vi "ParameterA.vi"(0 "VISA resource name":refnum<visa-resource-name>, 1 "Voltage Level (1.0)":dbl=1.0 min=0.005 max=20.0 format="%.3f", 2 "Integ Time (0: Short)":enum16{"SHORT", "MED/LONG"}(ring), 3 "Frequency (20)":dbl=20.0 min=20.0 max=1000000.0 format="%.2f", 5 "AT1":dbl=0.05 min=0.05 max=2.0 format="%.2f", 7 "Zone (0)":i8 min=0 max=3, 11 "error in (no error)":errorcluster, 12 "Impedance Z (10m)":dbl=0.01 min=0.01 max=100000000.0 format="%^.2e") -> (4 "VISA resource name out":refnum<visa-resource-name>, 8 "Parameter A":dbl format="%.2f", 15 "error out":errorcluster)   [LabVIEW 2015, in "Agilent 428X Series.lvlib"]
doc: "This Vi returns the value of parameter A.\n \n 5m 12m 0.1 0.15 \n---------------------------------------------------------------------------------------------------------\n A1=At1 * A1=At1 * A1=At1 \n A2=At1 A2=At1 A2=At2\nMed/Long A3=At1 A3=0.25 A3=0.25\n A4=At1 A4=At1 A4=At1\n---------------------------------------------------------------------------------------------------------\n 0.15 2 5 20 \n---------------------------------------------------------------------------------------------------------\n A1=At1 A1=At1 A1=At1 **\n A2=0.1 A2=At1 A2=At1\nMed/Long A3=0.25 A3=0.25 A3=0.25\n A4=0.1 A4=At1 A4=At1\n---------------------------------------------------------------------------------------------------------\n 5m 12m 0.1 0.15 \n---------------------------------------------------------------------------------------------------------\n A1=At1 A1=At1 A1=At1\nSHORT A2=At1 A2=At1 A2=0.1\n A3=At1 A3=0.25 A3=0.25\n A4=At1 A4=At1 A4=At1\n---------------------------------------------------------------------------------------------------------\n 0.15 2 5 20\n A1=At1 A1=At1 A1=At1 **\nSHORT A2=0.2 A2=At1 A2=At1\n A3=0.3 A3=0.3 A3=0.3\n A4=0.5*At1+0.1 A4=At1 A4=At1\n--------------------------------------------------------------------------------------------------------\n* : When test frewuency is less than 300Hz., 100Hz<=fm<=300Hz:\n Multiply the A values by 2. Fm<100Hz: Mulitply the A values by \n 2.5.\n**:Add 0.15 to the A values when all of the following measurement \n conditions are satisfied.\n Test Frequency: 300Hz<fm<=1MHz\n Test Signal Voltage: 5Vrms<Vs<=20Vrms\n DUT:Indicator,|Zm|<200Oohms\n\nDisclaimer: All accuracy calculation VI's are not part of the original \n driver. They are provided for supplementry purpose only.\n If user desires very high accuracy data, please do or \n check the calculation seperately."
uses:
  Agilent 428X Series.lvlib
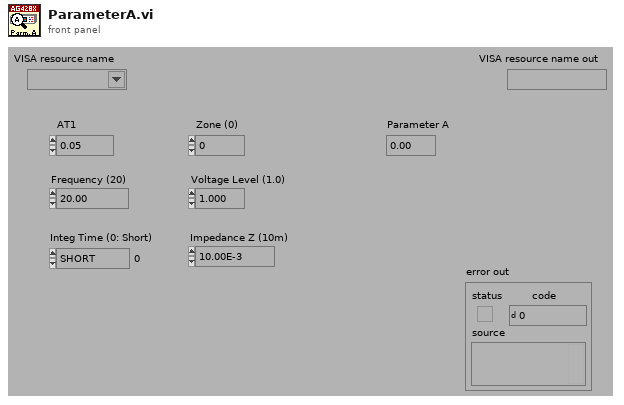
[diagram p1: front panel]
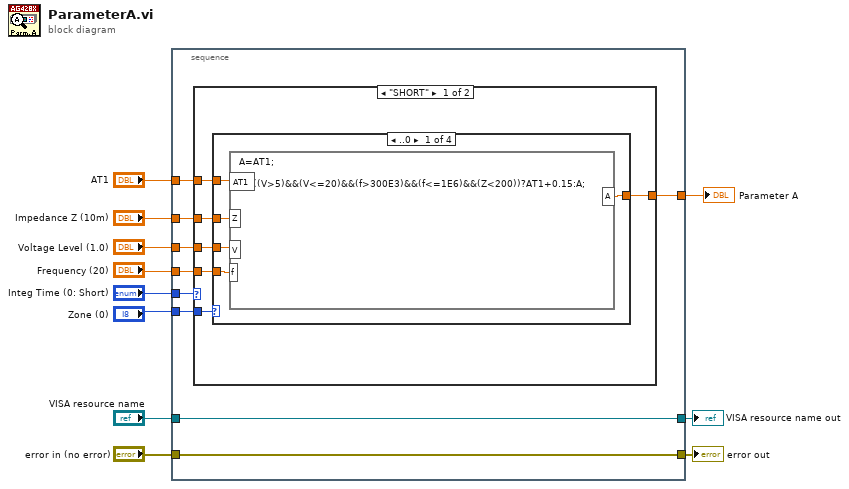
[diagram p0: block diagram]
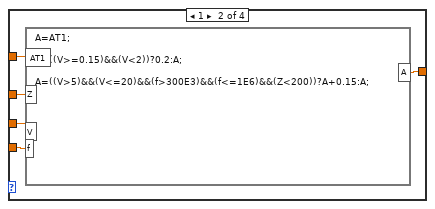
[diagram p2: hidden frame]
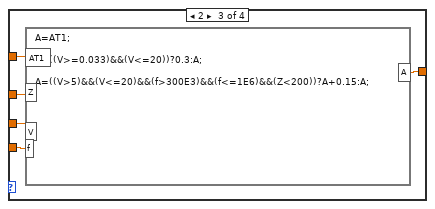
[diagram p3: hidden frame]
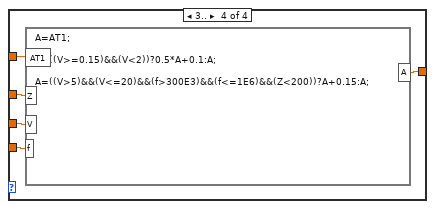
[diagram p4: hidden frame]
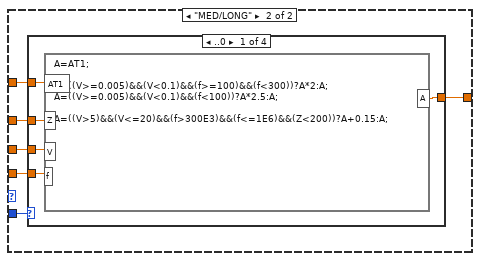
[diagram p5: hidden frame]
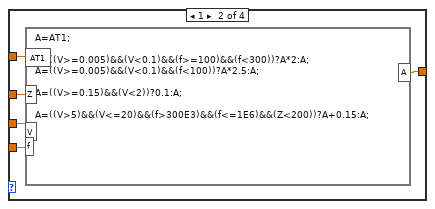
[diagram p6: hidden frame]
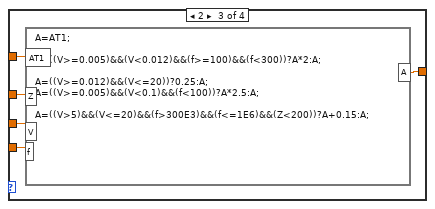
[diagram p7: hidden frame]
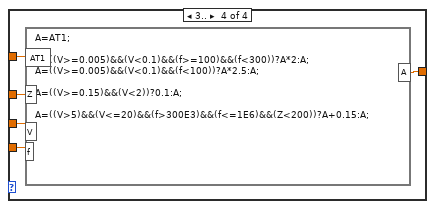
[diagram p8: hidden frame]
diagram:
  n1 = stacked-sequence {
    tunnel: "VISA resource name" -> [w20]
    tunnel: [w20] -> w10
    tunnel: "error in (no error)" -> [w19]
    tunnel: [w19] -> w8
    tunnel: "Zone (0)" -> [w18]
    tunnel: "AT1" -> [w17]
    tunnel: "Voltage Level (1.0)" -> [w16]
    tunnel: [w15] -> w4
    tunnel: "Integ Time (0: Short)" -> [w14]
    tunnel: "Frequency (20)" -> [w13]
    tunnel: "Impedance Z (10m)" -> [w12]
    frame #0 {
      n2 = case shown="\"SHORT\"" w14 {
        tunnel: [w26 w52] -> w15
        tunnel: w16 -> [w25 w51]
        tunnel: w17 -> [w24 w50]
        tunnel: w18 -> [w23 w49]
        tunnel: w13 -> [w22 w48]
        tunnel: w12 -> [w21 w47]
        frame "SHORT" {
          n3 = case shown="..0" w23 {
            tunnel: w24 -> [w31 w36 w41 w46]
            tunnel: w25 -> [w30 w35 w40 w45]
            tunnel: [w29 w34 w39 w44] -> w26
            tunnel: w22 -> [w28 w33 w38 w43]
            tunnel: w21 -> [w27 w32 w37 w42]
            frame ..0 {
              n4 = formula code="A=AT1;\n\nA=((V>5)&&(V<=20)&&(f>300E3)&&(f<=1E6)&&(Z<200))?AT1+0.15:A;"("AT1"=w31, "V"=w30, "f"=w28, "Z"=w27) -> ("A"=w29:dbl)
            }
            frame 1 {
              n5 = formula code="A=AT1;\n\nA=((V>=0.15)&&(V<2))?0.2:A;\n\nA=((V>5)&&(V<=20)&&(f>300E3)&&(f<=1E6)&&(Z<200))?A+0.15:A;"("AT1"=w36, "V"=w35, "f"=w33, "Z"=w32) -> ("A"=w34:dbl)
            }
            frame 2 {
              n6 = formula code="A=AT1;\n\nA=((V>=0.033)&&(V<=20))?0.3:A;\n\nA=((V>5)&&(V<=20)&&(f>300E3)&&(f<=1E6)&&(Z<200))?A+0.15:A;"("AT1"=w41, "V"=w40, "f"=w38, "Z"=w37) -> ("A"=w39:dbl)
            }
            frame 3.. {
              n7 = formula code="A=AT1;\n\nA=((V>=0.15)&&(V<2))?0.5*A+0.1:A;\n\nA=((V>5)&&(V<=20)&&(f>300E3)&&(f<=1E6)&&(Z<200))?A+0.15:A;"("AT1"=w46, "V"=w45, "f"=w43, "Z"=w42) -> ("A"=w44:dbl)
            }
          }
        }
        frame "MED/LONG" {
          n8 = case shown="..0" w49 {
            tunnel: w50 -> [w57 w62 w67 w72]
            tunnel: w51 -> [w56 w61 w66 w71]
            tunnel: [w55 w60 w65 w70] -> w52
            tunnel: w48 -> [w54 w58 w63 w68]
            tunnel: w47 -> [w53 w59 w64 w69]
            frame ..0 {
              n9 = formula code="A=AT1;\n\nA=((V>=0.005)&&(V<0.1)&&(f>=100)&&(f<300))?A*2:A;\nA=((V>=0.005)&&(V<0.1)&&(f<100))?A*2.5:A;\n\nA=((V>5)&&(V<=20)&&(f>300E3)&&(f<=1E6)&&(Z<200))?A+0.15:A;"("AT1"=w57, "V"=w56, "f"=w54, "Z"=w53) -> ("A"=w55:dbl)
            }
            frame 1 {
              n10 = formula code="A=AT1;\n\nA=((V>=0.005)&&(V<0.1)&&(f>=100)&&(f<300))?A*2:A;\nA=((V>=0.005)&&(V<0.1)&&(f<100))?A*2.5:A;\n\nA=((V>=0.15)&&(V<2))?0.1:A;\n\nA=((V>5)&&(V<=20)&&(f>300E3)&&(f<=1E6)&&(Z<200))?A+0.15:A;"("AT1"=w62, "V"=w61, "Z"=w59, "f"=w58) -> ("A"=w60:dbl)
            }
            frame 2 {
              n11 = formula code="A=AT1;\n\nA=((V>=0.005)&&(V<0.012)&&(f>=100)&&(f<300))?A*2:A;\n\nA=((V>=0.012)&&(V<=20))?0.25:A;\nA=((V>=0.005)&&(V<0.1)&&(f<100))?A*2.5:A;\n\nA=((V>5)&&(V<=20)&&(f>300E3)&&(f<=1E6)&&(Z<200))?A+0.15:A;"("AT1"=w67, "V"=w66, "Z"=w64, "f"=w63) -> ("A"=w65:dbl)
            }
            frame 3.. {
              n12 = formula code="A=AT1;\n\nA=((V>=0.005)&&(V<0.1)&&(f>=100)&&(f<300))?A*2:A;\nA=((V>=0.005)&&(V<0.1)&&(f<100))?A*2.5:A;\n\nA=((V>=0.15)&&(V<2))?0.1:A;\n\nA=((V>5)&&(V<=20)&&(f>300E3)&&(f<=1E6)&&(Z<200))?A+0.15:A;"("AT1"=w72, "V"=w71, "Z"=w69, "f"=w68) -> ("A"=w70:dbl)
            }
          }
        }
      }
    }
  }
  "error out" <- w8
  "VISA resource name out" <- w10
  "Parameter A" <- w4
